vi "SEH Execute Error Handling Code.vi"(8 "Internal Error In":errorcluster, 9 "Error to Process In":errorcluster, 11 "Code to Execute":string) -> (0 "Internal Error Out":errorcluster, 1 "Error to Process Out":errorcluster)   [LabVIEW 2014]
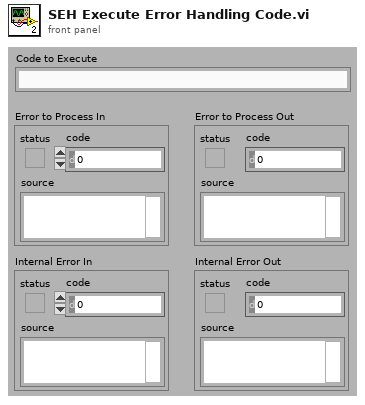
[diagram p1: front panel]
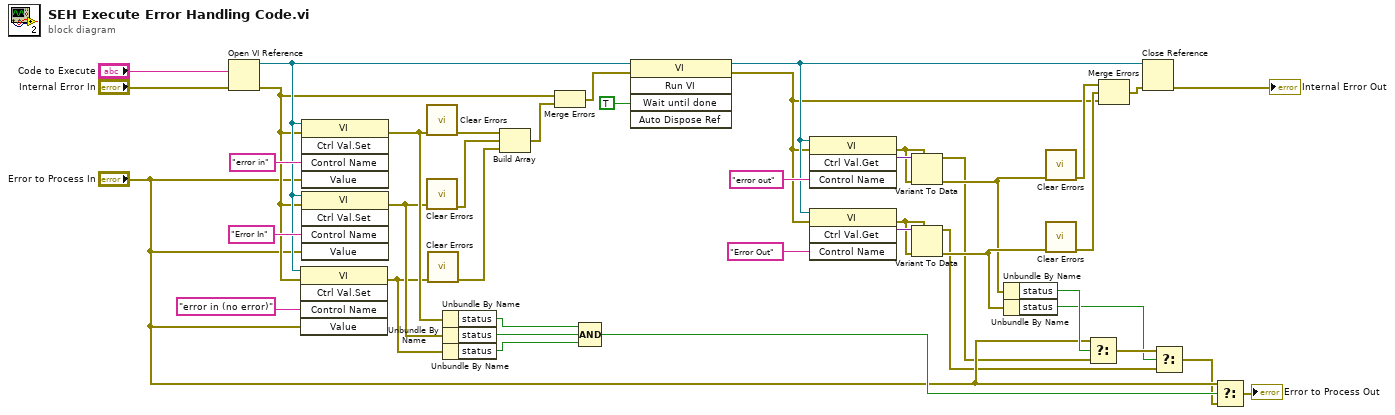
[diagram p0: block diagram]
diagram:
  n1 = Open VI Reference(vi path="Code to Execute", error in (no error)="Internal Error In") -> (vi reference=w17:refnum<vi>, error out=w16:errorcluster)  [unwired: 1 in, 3 out]
  n2 = invoke class="VI" method="Ctrl Val.Set"(reference=w17, error in=w16, "Control Name"="error in (no error)", "Value"="Error to Process In") -> (error out=w22:errorcluster)  [unwired: 1 in, 4 out]
  n3 = invoke class="VI" method="Ctrl Val.Set"(reference=w17, error in=w16, "Control Name"="error in", "Value"="Error to Process In") -> (error out=w29:errorcluster)  [unwired: 1 in, 4 out]
  n4 = invoke class="VI" method="Ctrl Val.Set"(reference=w17, error in=w16, "Control Name"="Error In", "Value"="Error to Process In") -> (error out=w28:errorcluster)  [unwired: 1 in, 4 out]
  n5 = call <vilib>:"Clear Errors.vi"("error in (no error)"=w29) -> ("error out"=w20:errorcluster)  [unwired: 1 in, 5 out]
  n6 = call <vilib>:"Clear Errors.vi"("error in (no error)"=w28) -> ("error out"=w19:errorcluster)  [unwired: 1 in, 5 out]
  n7 = call <vilib>:"Clear Errors.vi"("error in (no error)"=w22) -> ("error out"=w18:errorcluster)  [unwired: 1 in, 5 out]
  n8 = Unbundle By Name(w29) -> ("status"=w27:bool)
  n9 = Unbundle By Name(w28) -> ("status"=w26:bool)
  n10 = Unbundle By Name(w22) -> ("status"=w24:bool)
  n11 = Build Array(w20, w19, w18) -> (w21:errorcluster[])
  n12 = Merge Errors(w16, w21) -> (w40:errorcluster)
  n13 = Compound Arithmetic op=AND(w27, w26, w24) -> (w12:bool)
  n14 = invoke class="VI" method="Run VI"(reference=w17, error in=w40, "Wait until done"=TRUE ("Wait Until Done")) -> (reference out=w34:refnum<vi>, error out=w14:errorcluster)  [unwired: 2 in, 3 out]
  n15 = invoke class="VI" method="Ctrl Val.Get"(reference=w34, error in=w14, "Control Name"="error out") -> (error out=w6:errorcluster, "Get Control Value Variant"=w36:variant)  [unwired: 1 in, 2 out]
  n16 = invoke class="VI" method="Ctrl Val.Get"(reference=w34, error in=w14, "Control Name"="Error Out") -> (error out=w5:errorcluster, "Get Control Value Variant"=w35:variant)  [unwired: 1 in, 2 out]
  n17 = Variant To Data(error in=w6, type=w6, Variant=w36) -> (data=w3:errorcluster, error out=w15:errorcluster)
  n18 = Variant To Data(error in=w5, type=w5, Variant=w35) -> (data=w4:errorcluster, error out=w25:errorcluster)
  n19 = Unbundle By Name(w15) -> ("status"=w11:bool)
  n20 = Unbundle By Name(w25) -> ("status"=w8:bool)
  n21 = call <vilib>:"Clear Errors.vi"("error in (no error)"=w15) -> ("error out"=w33:errorcluster)  [unwired: 1 in, 5 out]
  n22 = call <vilib>:"Clear Errors.vi"("error in (no error)"=w25) -> ("error out"=w32:errorcluster)  [unwired: 1 in, 5 out]
  n23 = Select(t="Error to Process In", s=w11, f=w3) -> (s? t:f=w9:errorcluster)
  n24 = Merge Errors(w33, w32, w14) -> (w31:errorcluster)
  n25 = Close Reference(reference=w34, error in (no error)=w31) -> (error out=→"Internal Error Out":errorcluster)
  n26 = Select(t=w9, s=w8, f=w4) -> (s? t:f=w7:errorcluster)
  n27 = Select(t="Error to Process In", s=w12, f=w7) -> (s? t:f=→"Error to Process Out":errorcluster)
